vi "Main.vi"() -> ()   [LabVIEW 2016]
doc: "The myRIO Project template acquires acceleration data from the onboard accelerometer and displays the changes of acceleration values in a waveform chart."
uses:
  <vilib>/Platform/TimedLoop/XDataNode/timing_clust.ctl
  <vilib>/Platform/TimedLoop/XDataNode/nitl_modes.ctl
  <vilib>/Platform/TimedLoop/XDataNode/wakeup.ctl
  <vilib>/myRIO/Instrument Drivers/Onboard Devices/Accelerometer/typedefs/Accelerometer Reference.ctl
  <vilib>/myRIO/Common/Instrument Driver Framework/Utilities/typedefs/myRIO Generic Hardware Reference.ctl
  <vilib>/myRIO/Common/Instrument Driver Framework/Utilities/typedefs/Hardware Version Enum.ctl
  <vilib>/myRIO/Common/Instrument Driver Framework/Utilities/typedefs/myRIO v1.0 Reference.ctl
  <vilib>/myRIO/Common/Instrument Driver Framework/Utilities/typedefs/Generic FPGA Reference.ctl
  <vilib>/myRIO/Common/Instrument Driver Framework/myRIO v1.0/Accelerometer/typedefs/Accelerometer Channels List.ctl
  <vilib>/myRIO/Common/Instrument Driver Framework/myRIO v1.0/Accelerometer/typedefs/Accelerometer Channels Enum.ctl
  <vilib>/userdefined/High Color/nirio_resource_hc.ctl
  <vilib>/myRIO/Common/Instrument Driver Framework/Utilities/vis/Is FPGA Ref Available.vi
  <vilib>/myRIO/Common/Instrument Driver Framework/myRIO v1.0/Accelerometer/vis/myRIO v1.1 Open Accelerometer.vi
  <vilib>/myRIO/Instrument Drivers/Onboard Devices/Accelerometer/vis/Read.vi
  <vilib>/myRIO/Common/Instrument Driver Framework/Utilities/vis/Validate Channels.vi
  <vilib>/myRIO/Common/Instrument Driver Framework/myRIO v1.0/Accelerometer/vis/myRIO v1.0 Reserve Accelerometer.vi
  <vilib>/myRIO/Common/Instrument Driver Framework/myRIO v1.0/UART/vis/myRIO v1.0 Close UART.vi
  <vilib>/myRIO/Common/Instrument Driver Framework/myRIO v1.0/Resource Manager/vis/myRIO v1.0 Reserve Channel List.vi
  <vilib>/myRIO/Common/Instrument Driver Framework/myRIO v1.0/Accelerometer/vis/myRIO v1.0 Build MUX Configuration Accelerometer.vi
  <vilib>/myRIO/Common/Instrument Driver Framework/myRIO v1.0/Resource Manager/vis/myRIO v1.0 Reserve Channel.vi
  <vilib>/myRIO/Common/Instrument Driver Framework/myRIO v1.0/Resource Manager/vis/myRIO v1.0 Unreserve Channel.vi
  <vilib>/myRIO/Common/Instrument Driver Framework/myRIO v1.0/Resource Manager/vis/myRIO v1.0 Build Mutex Name.vi
  <vilib>/Utility/VariantDataType/GetNumericInfo.vi
  <vilib>/Utility/error.llb/Error Cluster From Error Code.vi
  <vilib>/myRIO/Common/Instrument Driver Framework/myRIO v1.0/myRIO v1.1 Open.vi
  <vilib>/myRIO/Common/Instrument Driver Framework/myRIO v1.0/Accelerometer/vis/myRIO v1.0 Get Scaling Constant Accelerometer.vi
  <vilib>/myRIO/Common/Instrument Driver Framework/Utilities/vis/IO Manager.vi
  <vilib>/myRIO/Common/Instrument Driver Framework/Utilities/vis/Configuration Manager.vi
  <vilib>/myRIO/Common/Instrument Driver Framework/myRIO v1.0/myRIO v1.0 Close.vi
  <vilib>/myRIO/Common/Instrument Driver Framework/myRIO v1.0/Accelerometer/vis/myRIO v1.0 Read Accelerometer.vi
  <vilib>/myRIO/Common/Instrument Driver Framework/Utilities/vis/FPGA Ref Manager.vi
  <vilib>/myRIO/Common/Instrument Driver Framework/myRIO v1.0/myRIO v1.0 Reset FPGA.vi
  <vilib>/myRIO/Common/Instrument Driver Framework/myRIO v1.0/IRQ/vis/myRIO v1.0 IRQ Info FGV.vi
  <vilib>/myRIO/Common/Instrument Driver Framework/myRIO v1.0/IRQ/vis/myRIO v1.0 Timer IRQ Info FGV.vi
  <vilib>/myRIO/Common/Instrument Driver Framework/myRIO v1.0/IRQ/vis/myRIO v1.0 ISR Agent.vi
  <vilib>/platform/TimedLoop/XDataNode/XDataNode.xnode
  <vilib>/myRIO/Express VI/Onboard Devices/Accelerometer/Accelerometer Express VI.xnode
  <vilib>/myRIO/Instrument Drivers/Onboard Devices/Accelerometer/vis/myRIO Accelerometer Open.xnode
  <vilib>/myRIO/Instrument Drivers/Utilities/Utilities.lvlib
  <vilib>/myRIO/Instrument Drivers/Onboard Devices/Accelerometer/Accelerometer.lvlib
  <vilib>/Platform/TimedLoop/XDataNode/XDNodeRunTimeDep.lvlib
panel:
  out "Acceleration":T1(graph)
  out "In case of Error":errorcluster
  in  "Stop":bool
  # "AIR MUSIC [Target End]"
  # "This VI is supposed to send accelerometer related data to the host PC where various algorithms are used to synthesize sound."
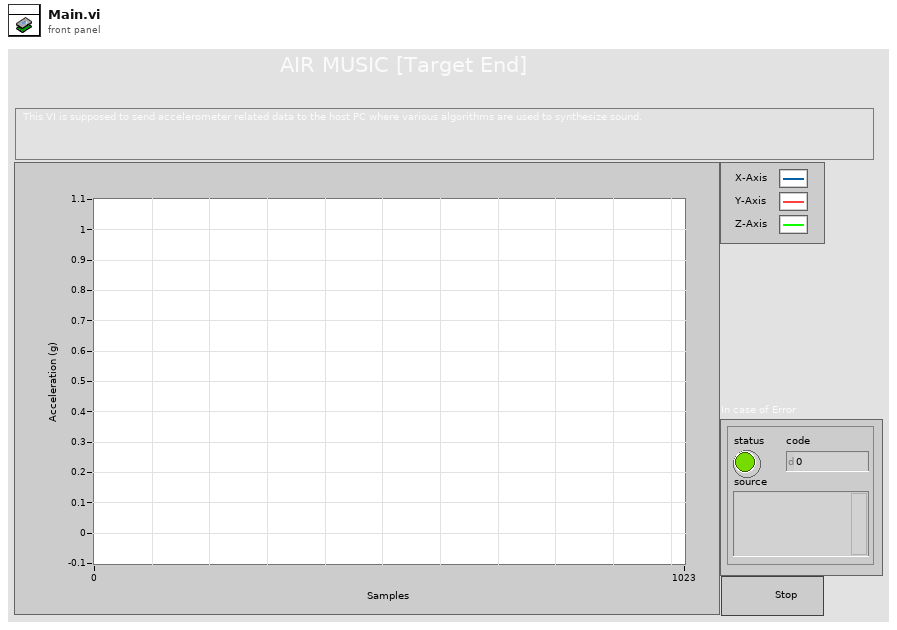
[diagram p1: front panel]
types:
  T1 = cluster{"X-Axis":dbl, "Y-Axis":dbl, "Z-Axis":dbl}
  T2 = typedef "XDNodeRunTimeDep.lvlib/timing_clust.ctl" = cluster{"Expected End [f-1]":u64, "Actual End [f-1]":u64, "Finished Late? [f-1]":bool, "Expected End [i-1]":u64, "Actual End [i-1]":u64, "Finished Late? [i-1]":bool, "Expected Start [i]":u64, "Actual Start [i]":u64, "Expected Start [f]":u64, "Actual Start [f]":u64, "Source Name":string, "Structure Name":string, "Period":i64, "Deadline":i64, "Offset":i64, "Start":i64, "Priority":i32, "Timeout":i32, "Mode":T3, "Wakeup Reason":T4, "Error":errorcluster, "Source Type":string, "Secondary Source Type":string, "Global End Time":u64, "Global Start Time":u64, "Frame Duration":u64, "Iteration Duration":u64, "Assigned CPU":i32, "I/O Scan Engine Mode":u32}
  T3 = typedef "XDNodeRunTimeDep.lvlib/nitl_modes.ctl" = enum32{"No Change", "Process missed periods, maintain original phase", "Discard missed periods, maintain original phase", "Process missed periods, ignore original phase", "Discard missed periods, ignore original phase"}
  T4 = typedef "XDNodeRunTimeDep.lvlib/wakeup.ctl" = enum32{"Normal", "Aborted", "Asynchronous wakeup", "Timing source error", "Timed loop error", "Timeout"}
  T5 = typedef "Accelerometer.lvlib/Accelerometer Reference.ctl" = cluster{"myRIO Reference":T6, "Accelerometer Channels List":T10, "LSB Weight":dbl}
  T6 = typedef "myRIO Generic Hardware Reference.ctl" = cluster{"myRIO Model":T7, "myRIO Hardware Reference":T8}
  T7 = typedef "Hardware Version Enum.ctl" = enum16{"Unknown", "myRIO-1900", "myRIO-1950", "roboRIO", "NI ELVIS RIO CM"}
  T8 = typedef "myRIO v1.0 Reference.ctl" = cluster{"Generic FPGA Reference":T9, "Allow multiple opens":bool}
  T9 = typedef "Generic FPGA Reference.ctl" = refnum<k20>
  T10 = typedef "Accelerometer Channels List.ctl" = T11[]
  T11 = typedef "Accelerometer Channels Enum.ctl" = enum16{"Not Connected", "X-Axis", "Y-Axis", "Z-Axis"}
  T12 = typedef "nirio_resource_hc.ctl" = tag
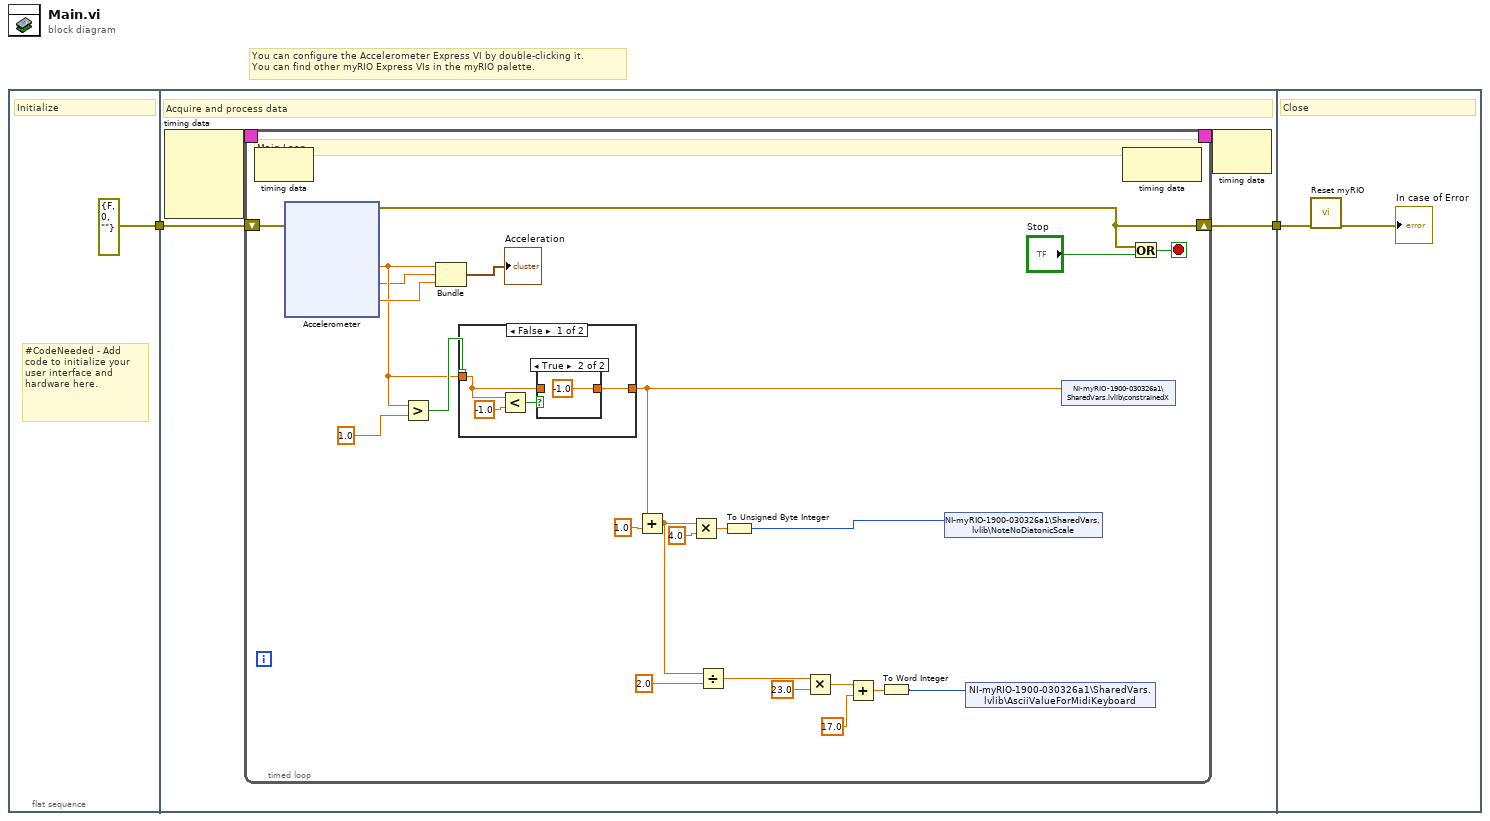
[diagram p0: block diagram]
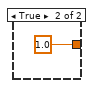
[diagram p3: hidden frame]
diagram:
  # "You can configure the Accelerometer Express VI by double-clicking it.\nYou can find other myRIO Express VIs in the myRIO palette."
  n1 = flat-sequence {
    tunnel: [errorcluster {"status"=FALSE, "code"=0, "source"=""} ("error in (no error)")] -> w2
    tunnel: w2 -> [w7]
    tunnel: [w6] -> w1
    tunnel: w1 -> [w82]
    frame #0 {
      # "#CodeNeeded - Add code to initialize your user interface and hardware here."
      # "Initialize"
    }
    frame #1 {
      # "Acquire and process data"
      n2 = node-c288() -> (w5:T2)  [unwired: 4 in]
      n3 = timed-loop {
        shift-right: [w26] -> w6
        shift-left: w7 -> [w27]
        timing: w5 -> [_]
        timing-out: [_] -> w4
        stop <- w29 stop-if-true
        # "Main Loop"
        n4 = node-c288() -> ()  [unwired: 1 in, 1 out]
        n5 = xnode "Accelerometer"("error in (no error)"=w27) -> ("X-Axis"=w22:dbl, "Y-Axis"=w16:dbl, "Z-Axis"=w25:dbl, "error out"=w26:errorcluster)
        n6 = Greater?(x=w22, y=1.0) -> (0:w23:bool)
        n7 = Bundle("X-Axis"=w22, "Y-Axis"=w16, "Z-Axis"=w25) -> (→"Acceleration":T1)  [unwired: 1 in]
        n8 = case shown="False" w23 {
          tunnel: [w33 1.0 ("y")] -> w18
          tunnel: w22 -> [w36 _]
          frame False {
            n9 = Less?(x=w36, y=-1.0) -> (x < y?=w34:bool)
            n10 = case shown="True" w34 {
              tunnel: w36 -> [w37 _]
              tunnel: [w37 -1.0 ("y")] -> w33
              frame False {
              }
              frame True {
              }
            }
          }
          frame True {
          }
        }
        n11 = Add(x=w18, y=1.0) -> (x+y=w15:dbl)
        n12 = Multiply(x=w15, y=4.0) -> (x*y=w21:dbl)
        n13 = Divide(x=w15, y=2.0) -> (x/y=w13:dbl)
        n14 = To Unsigned Byte Integer(number=w21) -> (unsigned 8bit integer=w17:u8)
        n15 = Multiply(x=w13, y=23.0) -> (x*y=w11:dbl)
        n16 = Add(x=w11, y=17.0) -> (x+y=w9:dbl)
        n17 = To Word Integer(number=w9) -> (16bit integer=w8:i16)
        n18 = shared-variable "NI-myRIO-1900-030326a1\\SharedVars.lvlib\\NoteNoDiatonicScale"(w17) -> ()  [unwired: 1 in, 1 out]
        n19 = shared-variable "NI-myRIO-1900-030326a1\\SharedVars.lvlib\\AsciiValueForMidiKeyboard"(w8) -> ()  [unwired: 1 in, 1 out]
        n20 = shared-variable "NI-myRIO-1900-030326a1\\SharedVars.lvlib\\constrainedX"(w18) -> ()  [unwired: 1 in, 1 out]
        n21 = node-c288() -> ()  [unwired: 1 in, 1 out]
        n22 = Or(x=w26, y="Stop") -> (x .or. y?=w29:bool)
      }
      n23 = node-c288(w4) -> ()  [unwired: 1 out]
    }
    frame #2 {
      # "Close"
      n24 = call <vilib>:"Reset myRIO.vi"("error in (no error)"=w82) -> ("error out"=→"In case of Error":errorcluster)  [unwired: 10 in]
    }
  }
